vi "Send check instructions.vi"(5 "version":string, 6 "current code":string, 7 "enabled codes":string, 8 "error in (no error)":errorcluster, 9 "prefix":string, 10 "instructions":string[](array[string]), 11 "Motor in":refnum<class "Motor.lvclass">) -> (0 "error out":errorcluster, 1 "error":bool, 2 "replies":string[](array[string]), 3 "Motor out":refnum<class "Motor.lvclass">, 4 "ok":bool)   [LabVIEW 2018, in "Motor.lvclass"]
uses:
  Motor.lvclass
  Motor.lvclass/Motor.ctl
panel:
  out "current time 2":timestamp format="%<%H:%M:%S%3u\n%Y/%m/%d>T"
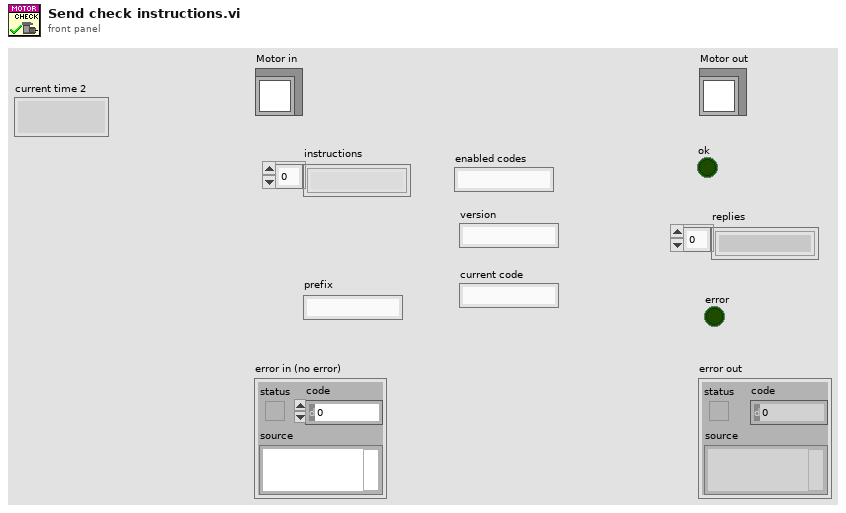
[diagram p1: front panel]
types:
  T1 = enum16{"Standard", "Buffered", "CRLF", "Immediate"}
  T2 = enum16{"open", "replace", "create", "open or create", "replace or create", "replace or create with confirmation"}
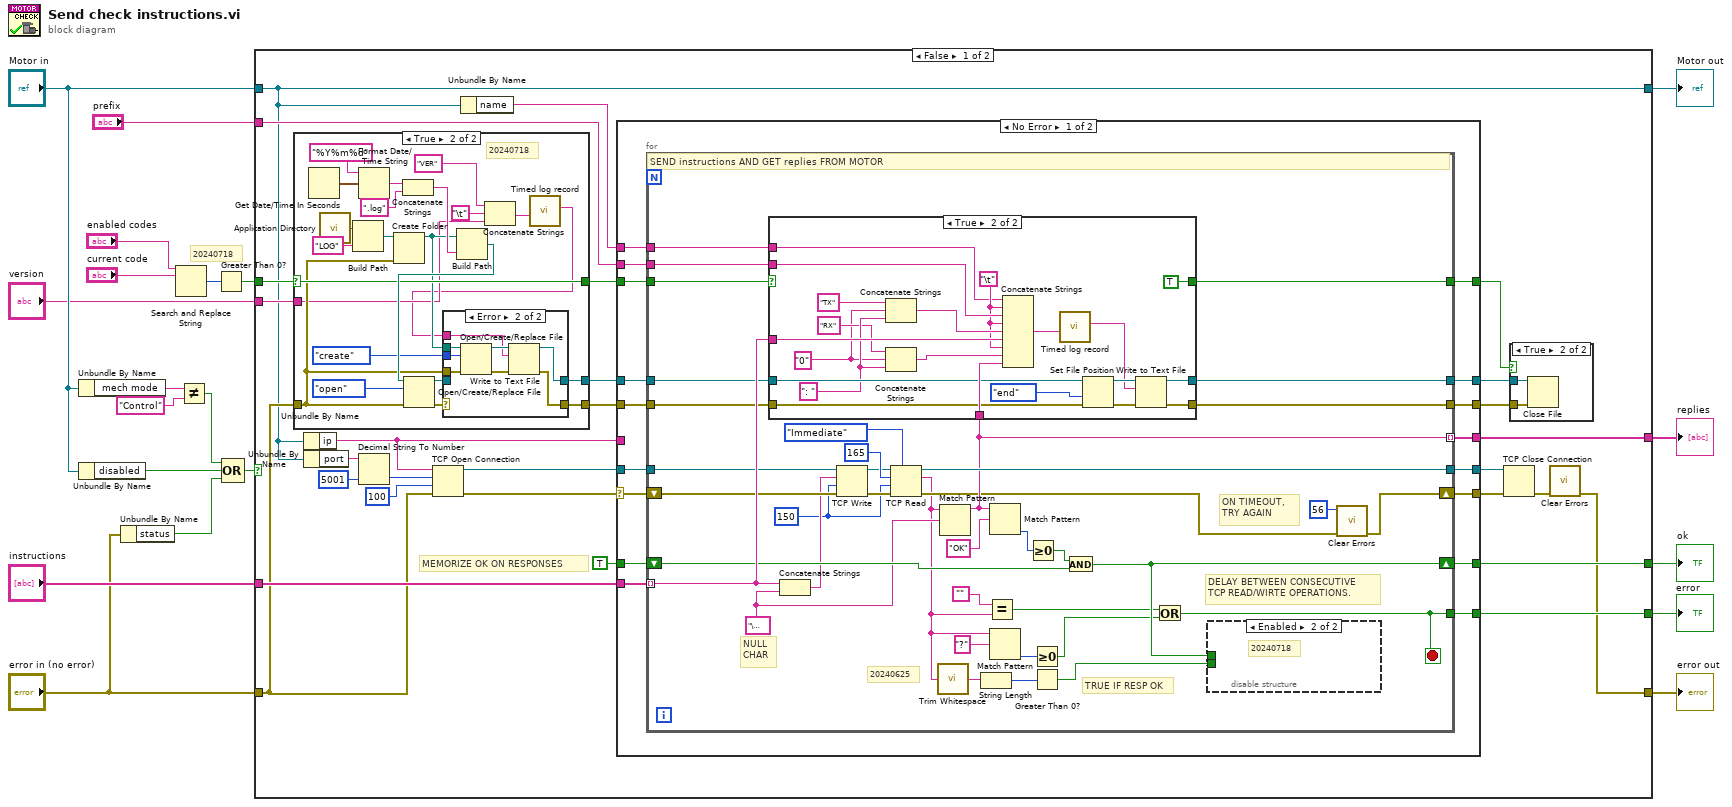
[diagram p0: block diagram]
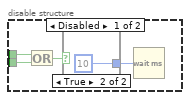
[diagram p2: hidden frame]
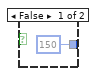
[diagram p3: hidden frame]
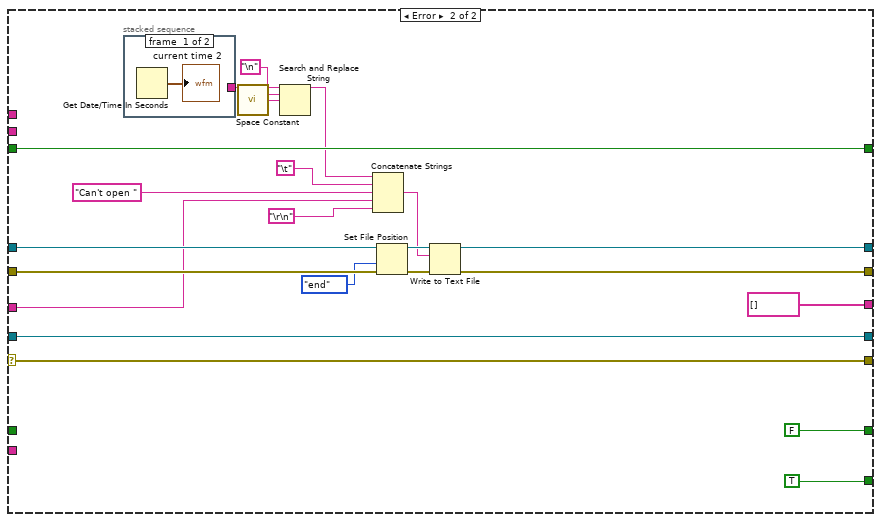
[diagram p5: hidden frame]
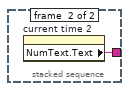
[diagram p6: hidden frame]
diagram:
  # "20240718"
  n1 = Unbundle By Name("Motor in") -> ("mech mode"=w13:string)
  n2 = Unbundle By Name("Motor in") -> ("disabled"=w10:bool)
  n3 = Unbundle By Name("error in (no error)") -> ("status"=w11:bool)
  n4 = Search and Replace String(input string="enabled codes", search string="current code") -> (number of replacements=w4:i32)  [unwired: 6 in, 3 out]
  n5 = Not Equal?(x=w13, y="Control") -> (x != y?=w7:bool)
  n6 = Greater Than 0?(x=w4) -> (x > 0?=w3:bool)
  n7 = Compound Arithmetic op=OR(w7, w10, w11) -> (w9:bool)
  n8 = case shown="False" w9 {
    tunnel: [w35 w195] -> w20
    tunnel: [w22 w196] -> w19
    tunnel: "Motor in" -> [w22 w196]
    tunnel: "instructions" -> [w44 _]
    tunnel: [w42 _] -> w17
    tunnel: [w38 _] -> w16
    tunnel: [w37 _] -> w15
    tunnel: "error in (no error)" -> [w31 w195]
    tunnel: w3 -> [w33 _]
    tunnel: "version" -> [w24 _]
    tunnel: "prefix" -> [w23 _]
    frame False {
      # "MEMORIZE OK ON RESPONSES"
      n9 = case shown="True" w33 {
        selector: w33 -> [w161 w174]
        tunnel: [w160 w172] -> w30
        tunnel: [_ w170] -> w34
        tunnel: [w161 w174] -> w32
        tunnel: w31 -> [w160 w169]
        tunnel: w24 -> [_ w165]
        frame False {
        }
        frame True {
          # "20240718"
          n10 = Get Date/Time In Seconds() -> (seconds since 1Jan1904=w180:timestamp)
          n11 = call <vilib>:"Application Directory.vi"() -> ("Application Directory"=w179:path)
          n12 = Build Path(base path=w179, name or relative path="LOG") -> (appended path=w184:path)
          n13 = Format Date/Time String(time format string (%c)="%Y%m%d", seconds (now)=w180) -> (date/time string=w181:string)  [unwired: 1 in]
          n14 = Create Folder(path (use dialog)=w184, error in=w169) -> (created path=w167:path)  [unwired: 1 in, 2 out]
          n15 = Concatenate Strings(w181, ".log" ("string")) -> (w183:string)
          n16 = Build Path(base path=w167, name or relative path=w183) -> (appended path=w182:path)
          n17 = Open/Create/Replace File(file path (use dialog)=w182, error in=w169, operation (0:open)=T2."open") -> (refnum out=w171:refnum<file>, error out=w173:errorcluster)  [unwired: 3 in, 1 out]
          n18 = Concatenate Strings("VER" ("string"), "\t", w165) -> (w163:string)
          n19 = call "Timed log record .vi"("log input"=w163) -> ("log register"=w162:string)  [unwired: 9 in, 1 out]
          n20 = case shown="Error" w173 {
            selector: w173 -> [w186 _]
            tunnel: [w186 w190] -> w172
            tunnel: w171 -> [w185 _]
            tunnel: [w185 w188] -> w170
            tunnel: w169 -> [_ w194]
            tunnel: T2."create" ("operation (0:open)") -> [_ w193]
            tunnel: w167 -> [_ w192]
            tunnel: w162 -> [_ w187]
            frame No Error {
            }
            frame Error {
              n21 = Open/Create/Replace File(file path (use dialog)=w192, error in=w194, operation (0:open)=w193) -> (refnum out=w189:refnum<file>, error out=w191:errorcluster)  [unwired: 3 in, 1 out]
              n22 = Write to Text File(file (use dialog)=w189, text=w187, error in=w191) -> (refnum out=w188:refnum<file>, error out=w190:errorcluster)  [unwired: 1 in, 1 out]
            }
          }
        }
      }
      n23 = Unbundle By Name(w22) -> ("ip"=w25:string)
      n24 = Unbundle By Name(w22) -> ("port"=w47:string)
      n25 = Decimal String To Number(string=w47, default (0L)=u16 5001 ("default (0 I32)")) -> (number=w45:u16)  [unwired: 1 in, 1 out]
      n26 = TCP Open Connection(address=w25, remote port or service name=w45, timeout ms (60000)=100, error in (no error)=w31) -> (connection ID=w43:refnum<k5>, error out=w26:errorcluster)  [unwired: 1 in]
      n27 = Unbundle By Name(w22) -> ("name"=w21:string)
      n28 = case shown="No Error" w26 {
        selector: w26 -> [w50 w153]
        tunnel: w44 -> [w65 _]
        tunnel: w43 -> [w64 w154]
        tunnel: [w63 TRUE] -> w42
        tunnel: TRUE -> [w62 _]
        tunnel: [w61 w154] -> w40
        tunnel: [w60 w153] -> w39
        tunnel: [w59 FALSE] -> w38
        tunnel: [w58 string[] []] -> w37
        tunnel: w34 -> [w57 w146]
        tunnel: w23 -> [w56 _]
        tunnel: w32 -> [w55 w155]
        tunnel: w30 -> [w54 w149]
        tunnel: [w53 w147] -> w29
        tunnel: [w52 w145] -> w28
        tunnel: [w51 w155] -> w27
        tunnel: w25 -> [_ w138]
        tunnel: w21 -> [w49 _]
        frame No Error {
          n29 = for {
            tunnel: w65 -> [w103] mode=indexing
            tunnel: w64 -> [w101]
            tunnel: [w96] -> w63
            shift-right: [w100] -> w59
            shift-left: w62 -> [w95]
            tunnel: [w99] -> w61
            shift-right: [w97] -> w60
            shift-left: w50 -> [w102]
            tunnel: [w98] -> w58 mode=indexing
            tunnel: w57 -> [w94]
            tunnel: w56 -> [w93]
            tunnel: w55 -> [w92]
            tunnel: w54 -> [w91]
            tunnel: [w90] -> w53
            tunnel: [w89] -> w52
            tunnel: [w88] -> w51
            tunnel: w49 -> [w87]
            stop <- w96 stop-if-true
            w81 = 150 ("timeout ms (60000)")
            w77 = "\u0000" ("search string")
            # "DELAY BETWEEN CONSECUTIVE\nTCP READ/WIRTE OPERATIONS."
            # "ON TIMEOUT, TRY AGAIN"
            # "20240625"
            # "TRUE IF RESP OK"
            # "NULL\nCHAR"
            # "SEND instructions AND GET replies FROM MOTOR"
            n30 = Concatenate Strings(w103, w77) -> (w82:string)
            n31 = TCP Write(connection ID=w101, data in=w82, error in (no error)=w102, 9:w81) -> (connection ID out=w84:refnum<k5>, error out=w86:errorcluster)  [unwired: 1 out]
            n32 = TCP Read(connection ID=w84, bytes to read=165, error in (no error)=w86, 7:T1."Immediate" ("mode (standard)"), 9:w81) -> (connection ID out=w99:refnum<k5>, data out=w69:string, error out=w71:errorcluster)
            n33 = call <vilib>:"Trim Whitespace.vi"("string"=w69) -> ("trimmed string"=w68:string)  [unwired: 1 in]
            n34 = Match Pattern(string=w69, regular expression=w77) -> (before substring=w98:string)  [unwired: 1 in, 3 out]
            n35 = case shown="True" w92 {
              selector: w92 -> [w110 _]
              tunnel: w93 -> [_ w118]
              tunnel: w98 -> [_ w133]
              tunnel: w103 -> [_ w132]
              tunnel: w94 -> [w112 w130]
              tunnel: w91 -> [w111 w129]
              tunnel: [w111 w126] -> w90
              tunnel: [w112 w125] -> w89
              tunnel: [w110 TRUE] -> w88
              tunnel: w87 -> [_ w116]
              frame False {
              }
              frame True {
                w113 = "0"
                w122 = ": "
                w117 = "\t"
                n36 = Concatenate Strings("TX", w113, w122) -> (w119:string)
                n37 = Concatenate Strings("RX", w113, w122) -> (w120:string)
                n38 = Concatenate Strings(w116, w117, w118, w117, w119, w132, w117, w120, w133) -> (w115:string)
                n39 = call "Timed log record .vi"("log input"=w115) -> ("log register"=w114:string)  [unwired: 9 in, 1 out]
                n40 = Set File Position(refnum=w130, from (0:start)=enum16{"start", "end", "current"}."end", error in=w129) -> (refnum out=w127:refnum<file>, error out=w128:errorcluster)  [unwired: 1 in]
                n41 = Write to Text File(file (use dialog)=w127, text=w114, error in=w128) -> (refnum out=w125:refnum<file>, error out=w126:errorcluster)  [unwired: 1 in, 1 out]
              }
            }
            n42 = String Length(string=w68) -> (length=w67:i32)
            n43 = Equal?(x="", y=w69) -> (x = y?=w73:bool)
            n44 = Match Pattern(string=w98, regular expression="OK" ("y")) -> (offset past match=w76:i32)  [unwired: 1 in, 3 out]
            n45 = Match Pattern(string=w69, regular expression="?") -> (offset past match=w80:i32)  [unwired: 1 in, 3 out]
            n46 = Greater Or Equal To 0?(x=w76) -> (x >= 0?=w75:bool)
            n47 = Greater Or Equal To 0?(x=w80) -> (x >= 0?=w74:bool)
            n48 = Greater Than 0?(x=w67) -> (x > 0?=w66:bool)
            n49 = And(x=w75, y=w95) -> (x .and. y?=w100:bool)
            n50 = Or(x=w73, y=w74) -> (x .or. y?=w96:bool)
            n51 = disable-structure shown="Enabled" {
              disable-tunnel: w100 -> [w107 _]
              disable-tunnel: w66 -> [w104 _]
              frame Disabled {
                n52 = Or(x=w107, y=w104) -> (x .or. y?=w106:bool)
                n53 = case shown="True" w106 {
                  tunnel: [u32 150 ("milliseconds to wait") u32 10 ("milliseconds to wait")] -> w105
                  frame False {
                  }
                  frame True {
                  }
                }
                n54 = Wait (ms)(milliseconds to wait=w105) -> ()  [unwired: 1 out]
              }
              frame Enabled {
                # "20240718"
              }
            }
            n55 = call <vilib>:"Clear Errors.vi"("error in (no error)"=w71, "specific error code to clear (0: all)"=56) -> ("error out"=w97:errorcluster)  [unwired: 4 in, 1 out]
          }
        }
        frame Error {
          n56 = stacked-sequence {
            tunnel: [_ w157] -> w142
            frame #0 {
              n57 = Get Date/Time In Seconds() -> (seconds since 1Jan1904=→"current time 2":timestamp)
            }
            frame #1 {
              n58 = property on="current time 2" class="AbsTime (strict)"() -> ("NumText.Text"=w157:string)  [unwired: 2 in, 2 out]
            }
          }
          n59 = call <vilib>:"Space Constant.vi"() -> ("String"=w141:string)
          n60 = Search and Replace String(input string=w142, search string="\n", replace string=w141) -> (result string=w136:string)  [unwired: 5 in, 3 out]
          n61 = Concatenate Strings(w136, "\t", "Can't open " ("string"), w138, "\r\n") -> (w144:string)
          n62 = Set File Position(refnum=w146, from (0:start)=enum16{"start", "end", "current"}."end", error in=w149) -> (refnum out=w150:refnum<file>, error out=w148:errorcluster)  [unwired: 1 in]
          n63 = Write to Text File(file (use dialog)=w150, text=w144, error in=w148) -> (refnum out=w145:refnum<file>, error out=w147:errorcluster)  [unwired: 1 in, 1 out]
        }
      }
      n64 = TCP Close Connection(connection ID=w40, error in (no error)=w39) -> (error out=w36:errorcluster)  [unwired: 1 in, 1 out]
      n65 = case shown="True" w27 {
        tunnel: w29 -> [_ w159]
        tunnel: w28 -> [_ w158]
        frame False {
        }
        frame True {
          n66 = Close File(refnum=w158, error in=w159) -> ()  [unwired: 2 out]
        }
      }
      n67 = call <vilib>:"Clear Errors.vi"("error in (no error)"=w36) -> ("error out"=w35:errorcluster)  [unwired: 5 in, 1 out]
    }
    frame True {
    }
  }
  "error out" <- w20
  "Motor out" <- w19
  "error" <- w17
  "ok" <- w16
  "replies" <- w15
